vi "UDP Data Link - Configuration Utilities - Set Local IP Address State.vi"(8 "error in (no error)":errorcluster, 10 "State":T1(ring), 11 "Item Ref in":T2 format="%.0x") -> (0 "error out":errorcluster, 3 "Item Ref out":T2 format="%.0x")   [LabVIEW 2015, in "UDP Data Link System Explorer.lvlib"]
uses:
  UDP Data Link System Explorer.lvlib
  <vilib>/NI Veristand/Custom Device API/Custom Device Item Ref.ctl
  Shared/UDP Data Link Global.vi
  <vilib>/NI Veristand/Custom Device API/Set Item Property (Variant).vi
  Shared/UDP Data Link Shared.lvlib
  <vilib>/NI Veristand/Custom Device API/Custom Device API.lvlib
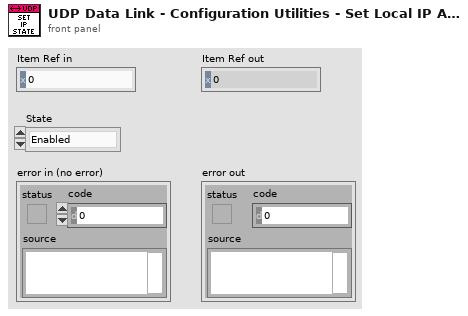
[diagram p1: front panel]
types:
  T1 = enum8{"Enabled", "Disabled", "Disabled and Grayed Out"}
  T2 = typedef "Custom Device API.lvlib/Custom Device Item Ref.ctl" = u64
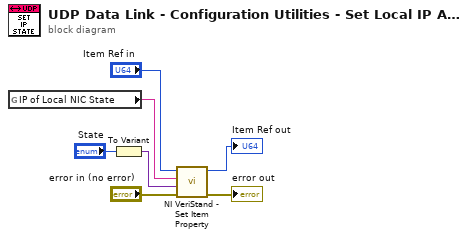
[diagram p0: block diagram]
diagram:
  n1 = global read "UDP Data Link Global.vi" "IP of Local NIC State"() -> (w5:string)
  n2 = To Variant(anything="State") -> (Variant=w1:variant)
  n3 = call-poly <vilib>:"NI VeriStand - Set Item Property.vi"("error in (no error)"="error in (no error)", "Value"=w1, "Property Name"=w5, "Item Ref in"="Item Ref in") -> ("error out"=→"error out":errorcluster, "Item Ref out"=→"Item Ref out":T2)  [unwired: 5 in, 1 out]
